vi "DAQmx Read (Digital 1D Bool NChan 1Samp 1Line).vi"(0 "task/channels in":refnum<k21>, 9 "timeout":dbl=10.0 format="%0.2f", 11 "error in":errorcluster) -> (4 "task out":refnum<k21>, 6 "data":bool[](array[boolean]), 15 "error out":errorcluster)   [LabVIEW 2011]
doc: "Reads a single Boolean sample from each channel in a task that contains one or more digital input channels. Each channel must contain only a single digital line."
uses:
  nilvaiu.dll
panel:
  # "channel"
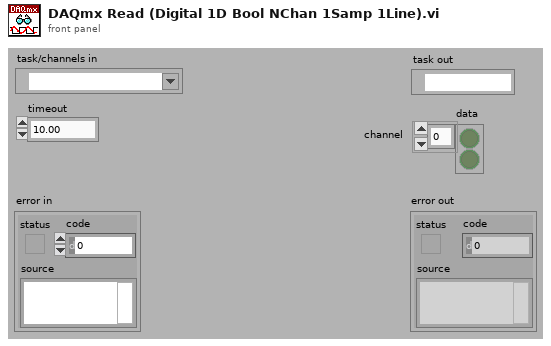
[diagram p1: front panel]
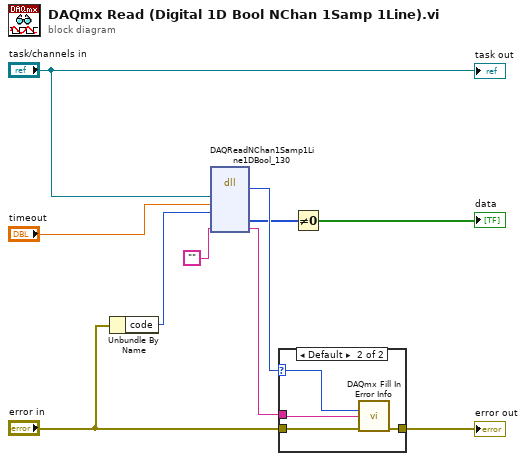
[diagram p0: block diagram]
diagram:
  n1 = Unbundle By Name("error in") -> ("code"=w1:i32)
  n2 = dll-call lib="nilvaiu.dll" fn="DAQReadNChan1Samp1Line1DBool_130"("taskID"="task/channels in", "timeout"="timeout", "incomingStatus"=w1, "extendedErrorInfo"="") -> (w7:i32, "data"=w3:u8[], "extendedErrorInfo"=w5:string)  [unwired: 6 in, 3 out]
  n3 = case shown="Default" w7 {
    selector: w7 -> [_ w14]
    tunnel: "error in" -> [w11 w15]
    tunnel: [w11 w13] -> w10
    tunnel: w5 -> [_ w12]
    frame 0 {
    }
    frame Default {
      n4 = call "DAQmx Fill In Error Info.vi"("status code"=w14, "extended error info"=w12, "error in"=w15) -> ("error out"=w13:errorcluster)  [unwired: 1 in, 11 out]
    }
  }
  "error out" <- w10
  n5 = Not Equal To 0?(x=w3) -> (x != 0?=→"data":bool[])
  "task out" <- "task/channels in"
